vi "Timer.vi"(0 "Wait_Time":dbl=10.0 format="%#_13g", 11 "Error_In":errorcluster, 13 "Timer_Operation_Select":T1=enum."Time_Out?") -> (4 "Time_Out?":bool, 6 "Start?":bool, 8 "Time":dbl, 15 "Error_Out":errorcluster)   [LabVIEW 2021]
doc: "Used as a typical timer."
uses:
  Controls/Timer_Data.ctl
  Controls/Timer_Operation_Select.ctl
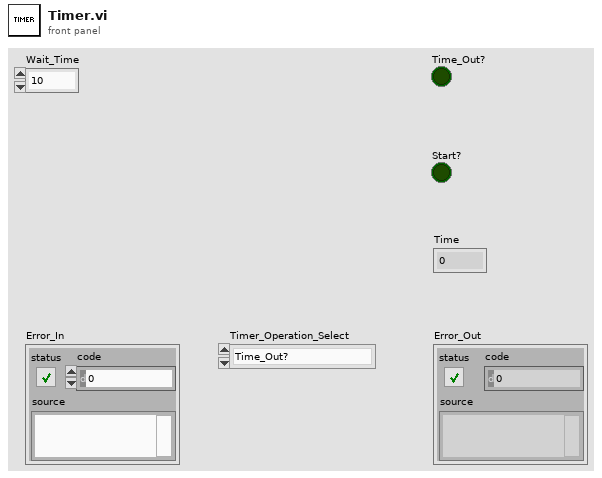
[diagram p1: front panel]
types:
  T1 = typedef "Timer_Operation_Select.ctl" = enum16{"Start_Timer", "Time_Out?", "Pause_Timer", "Stop_Timer"}
  T2 = typedef "Timer_Data.ctl" = cluster{"Start_Time":dbl, "Start?":bool, "Wait_Time":dbl, "Time":dbl}
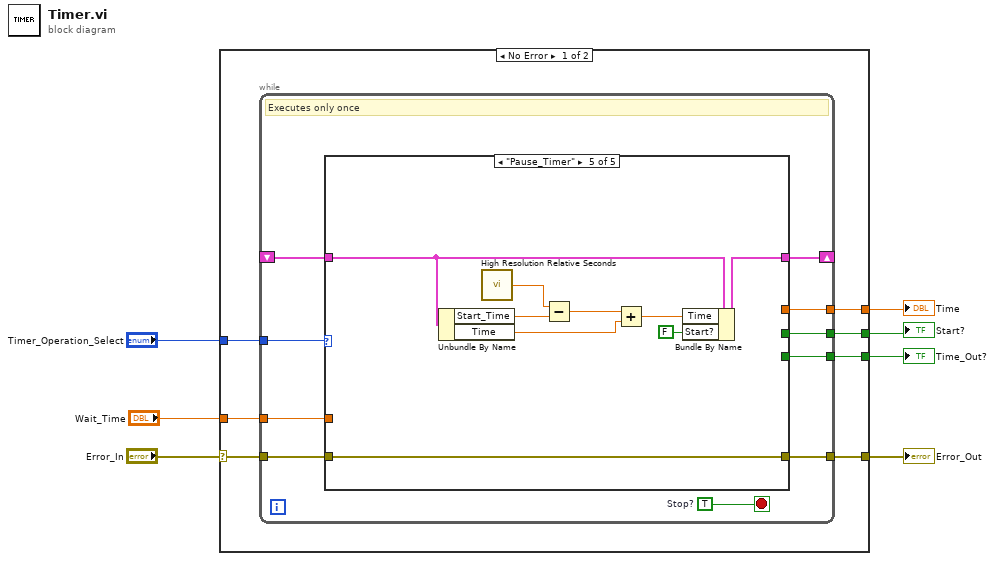
[diagram p0: block diagram]
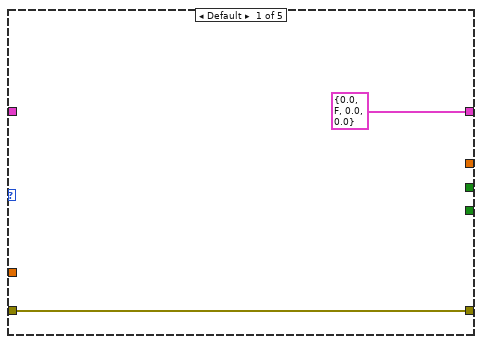
[diagram p2: hidden frame]
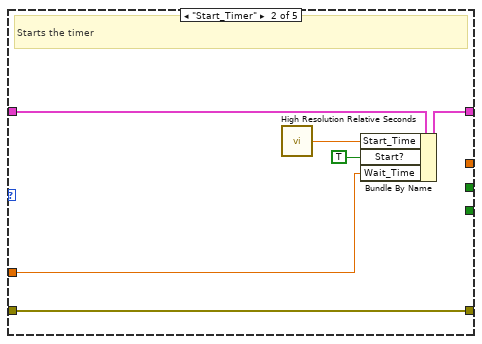
[diagram p3: hidden frame]
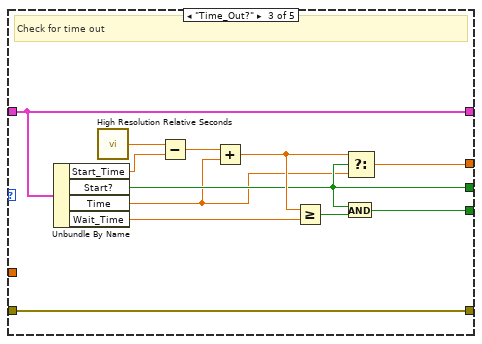
[diagram p4: hidden frame]
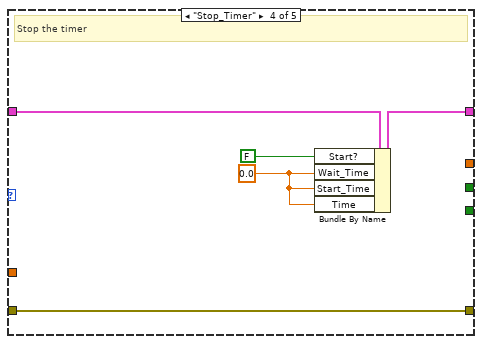
[diagram p5: hidden frame]
diagram:
  n1 = case shown="No Error" "Error_In" {
    selector: "Error_In" -> [w10 w59]
    tunnel: [w14 _] -> w7
    tunnel: [w13 w59] -> w6
    tunnel: "Wait_Time" -> [w12 _]
    tunnel: "Timer_Operation_Select" -> [w11 _]
    tunnel: [w9 _] -> w2
    tunnel: [w8 _] -> w1
    frame No Error {
      n2 = while {
        tunnel: w11 -> [w24]
        shift-right: [w23] -> _
        shift-left: _ -> [w22]
        tunnel: [w21] -> w14
        tunnel: w10 -> [w19]
        tunnel: [w18] -> w13
        tunnel: w12 -> [w17]
        tunnel: [w16] -> w9
        tunnel: [w15] -> w8
        stop <- w20 stop-if-true
        w20 = TRUE  # Stop?
        # "Executes only once"
        n3 = case shown="\"Pause_Timer\"" w24 {
          tunnel: [T2 {"Start_Time"=0.0, "Start?"=FALSE, "Wait_Time"=0.0, "Time"=0.0} ("Cluster") w30 w39 w47 w57] -> w23
          tunnel: w22 -> [_ w31 w39 w48 w56]
          tunnel: [_ _ w40 _ _] -> w21
          tunnel: w19 -> [w26 w32 w42 w49 w58]
          tunnel: [w26 w32 w42 w49 w58] -> w18
          tunnel: w17 -> [_ w27 _ _ _]
          tunnel: [_ _ w35 _ _] -> w16
          tunnel: [_ _ w33 _ _] -> w15
          frame Default {
          }
          frame "Start_Timer" {
            # "Starts the timer"
            n4 = call <vilib>:"High Resolution Relative Seconds.vi"() -> ("relative seconds"=w29:dbl)
            n5 = Bundle By Name(cluster=w31, "Start_Time"=w29, "Start?"=TRUE, "Wait_Time"=w27) -> (w30:T2)
          }
          frame "Time_Out?" {
            # "Check for time out"
            n6 = Unbundle By Name(w39) -> ("Start_Time"=w38:dbl, "Start?"=w35:bool, "Time"=w34:dbl, "Wait_Time"=w37:dbl)
            n7 = call <vilib>:"High Resolution Relative Seconds.vi"() -> ("relative seconds"=w41:dbl)
            n8 = Subtract(x=w41, y=w38) -> (x-y=w44:dbl)
            n9 = Add(x=w44, y=w34) -> (x+y=w36:dbl)
            n10 = Greater Or Equal?(x=w36, y=w37) -> (x >= y?=w43:bool)
            n11 = And(x=w35, y=w43) -> (x .and. y?=w40:bool)
            n12 = Select(t=w36, s=w35, f=w34) -> (s? t:f=w33:dbl)
          }
          frame "Stop_Timer" {
            w45 = 0.0 ("Wait_Time")
            # "Stop the timer"
            n13 = Bundle By Name(cluster=w48, "Start?"=FALSE, "Wait_Time"=w45, "Start_Time"=w45, "Time"=w45) -> (w47:T2)
          }
          frame "Pause_Timer" {
            n14 = Unbundle By Name(w56) -> ("Start_Time"=w55:dbl, "Time"=w50:dbl)
            n15 = call <vilib>:"High Resolution Relative Seconds.vi"() -> ("relative seconds"=w54:dbl)
            n16 = Subtract(x=w54, y=w55) -> (x-y=w53:dbl)
            n17 = Add(x=w53, y=w50) -> (x+y=w51:dbl)
            n18 = Bundle By Name(cluster=w56, "Time"=w51, "Start?"=FALSE) -> (w57:T2)
          }
        }
      }
    }
    frame Error {
    }
  }
  "Time_Out?" <- w7
  "Error_Out" <- w6
  "Start?" <- w2
  "Time" <- w1
